vi "Main_State_Calibrate_Position_2.vi"(0 "Motor Position Encoder [deg]":dbl=10.044943820224718 format="%#.3f", 1 "Motor Position Encoder Offset [deg]":dbl caption="Encoder Offset [deg]" format="%#.3f", 5 "Motor Velocity Encoder [deg/s]":dbl format="%#.3f", 7 "Period (Control Loop) [s]":dbl=0.001 caption="Period [s]", 9 "Motor Current Monitor [A]":dbl=-0.009079300589999995, 11 "Requested State":T3, 12 "PID Settings":T1={"Gains"={"K(e)"=0.0, "Kp"=0.8, "Ki"=0.0, "Kd"=0.003}, "Non-linear gain"={"Non-linear gain P"=enum."off", "Non-linear gain I"=enum."off", "Non-linear gain D"=enum."off"}, "D-Part variable"=enum."process variable", "Velocity estimate dy/dt"=enum."external", "Anti reset windup"=TRUE, "I-Part error band"=inf}, 13 "Current Settings":T2={"CW Current Threshold [A]"=0.5, "CCW Current Threshold [A]"=-0.5, "CW Output Range [A]"={"output high"=0.6, "output low"=0.0}, "CCW Output Range [A]"={"output high"=0.0, "output low"=-0.6}}, 14 "Reset?":bool) -> (3 "New Motor Position Encoder Offset [deg]":dbl caption="Encoder Offset [deg]" format="%#.3f", 4 "Velocity Setpoint [deg/s]":dbl, 6 "Command Variable u [A]":dbl, 10 "Calibration Finished?":bool, 15 "New Desired State":T3)   [LabVIEW 2015]
uses:
  Shared TypeDefs/Enum_Robot_States.ctl
  PID_Settings.ctl
  Enum_States_Calibrate_Position.ctl
  <vilib>/addons/control/pid/NI_PID_pid.lvlib
  <vilib>/ptbypt/NI_PtbyPt.lvlib
panel:
  out "Motor Position Encoder ROM CCW [deg]":dbl=10.044943820224718 format="%#_13g"
  out "Motor Position Encoder ROM CW [deg]":dbl=10.044943820224718 format="%#_13g"
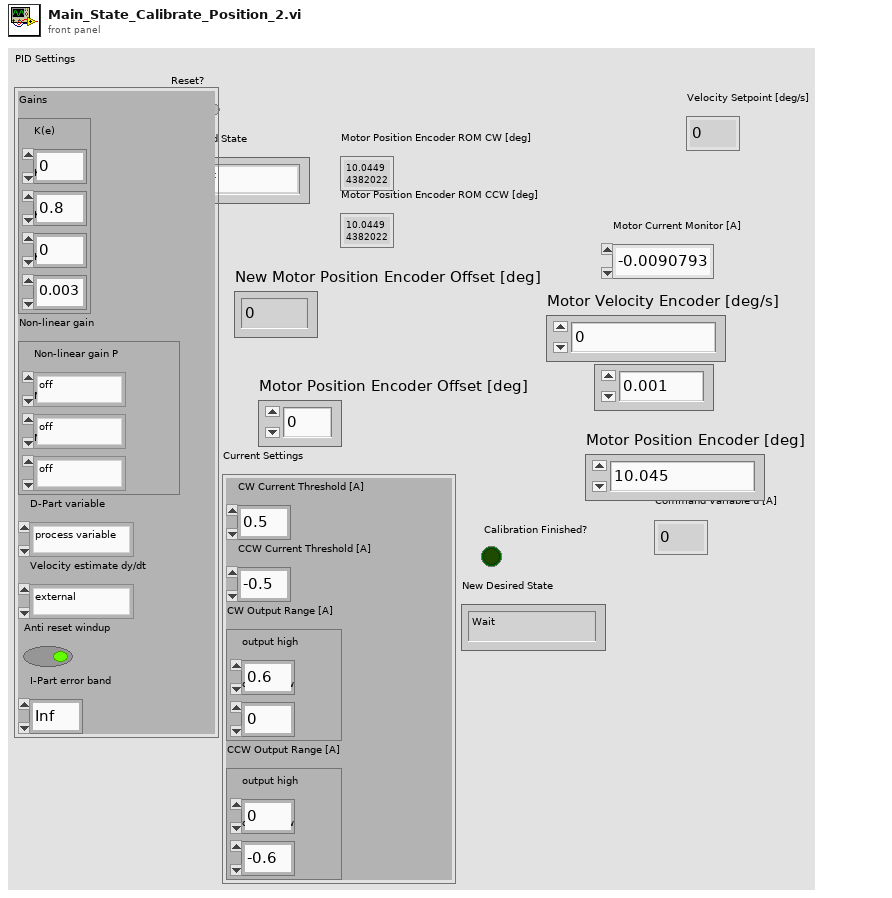
[diagram p1: front panel]
types:
  T1 = typedef "PID_Settings.ctl" = cluster{"Gains":cluster{"K(e)":sgl, "Kp":sgl, "Ki":sgl, "Kd":sgl}, "Non-linear gain":cluster{"Non-linear gain P":enum8{"exponential", "quadratic", "off"}, "Non-linear gain I":enum8{"exponential", "quadratic", "off"}, "Non-linear gain D":enum8{"exponential", "quadratic", "off"}}, "D-Part variable":enum8{"error", "process variable"}, "Velocity estimate dy/dt":enum8{"derivative", "external"}, "Anti reset windup":bool, "I-Part error band":sgl}
  T2 = cluster{"CW Current Threshold [A]":dbl, "CCW Current Threshold [A]":dbl, "CW Output Range [A]":cluster{"output high":dbl, "output low":dbl}, "CCW Output Range [A]":cluster{"output high":dbl, "output low":dbl}}
  T3 = typedef "Enum_Robot_States.ctl" = enum8{"Wait", "Reset", "Calibrate Position", "Calibrate Static Friction", "Hold", "Move (minJerk)", "PID Tuning", "Static Friction Measurement", "Dynamic Friction Measurement"}
  T4 = typedef "Enum_States_Calibrate_Position.ctl" = enum8{"Find Wall CW", "Find Wall CCW"}
  T5 = cluster{"K(e)":sgl, "Kp":sgl, "Ki":sgl, "Kd":sgl}
  T6 = cluster{"Non-linear gain P":enum8{"exponential", "quadratic", "off"}, "Non-linear gain I":enum8{"exponential", "quadratic", "off"}, "Non-linear gain D":enum8{"exponential", "quadratic", "off"}}
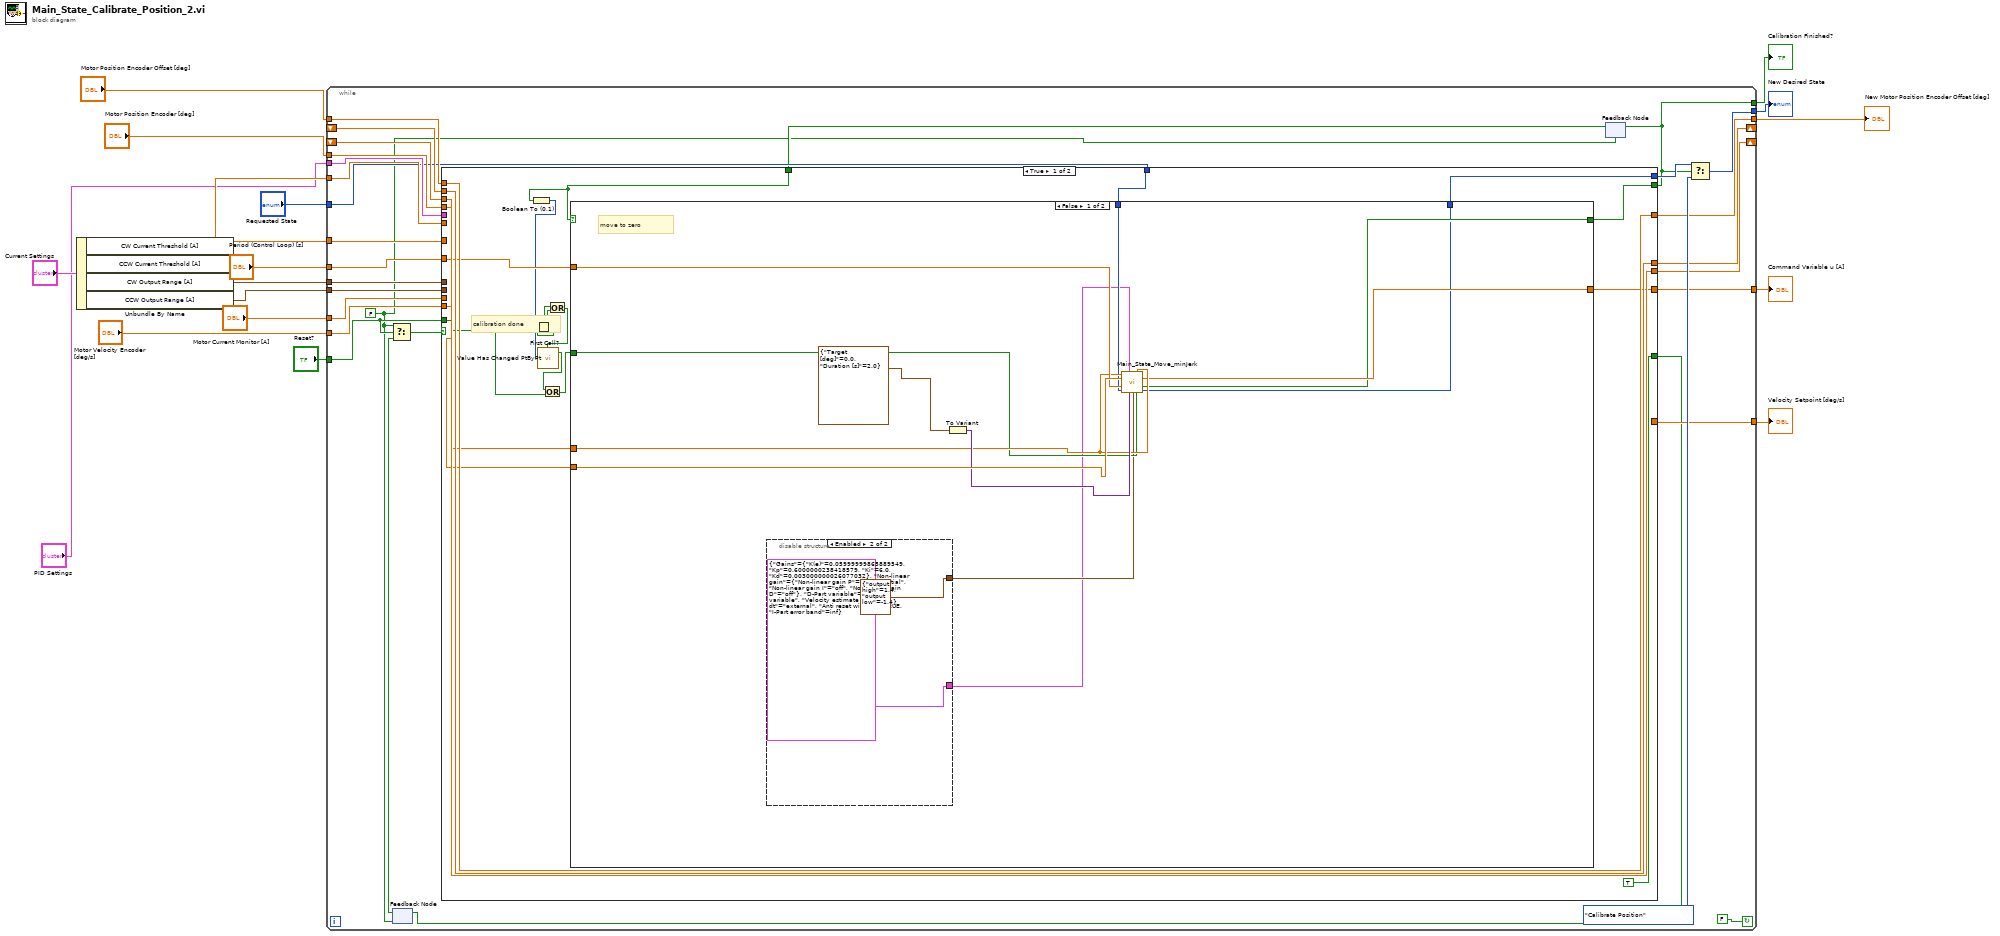
[diagram p0: block diagram]
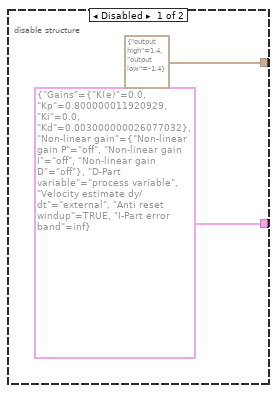
[diagram p2: hidden frame]
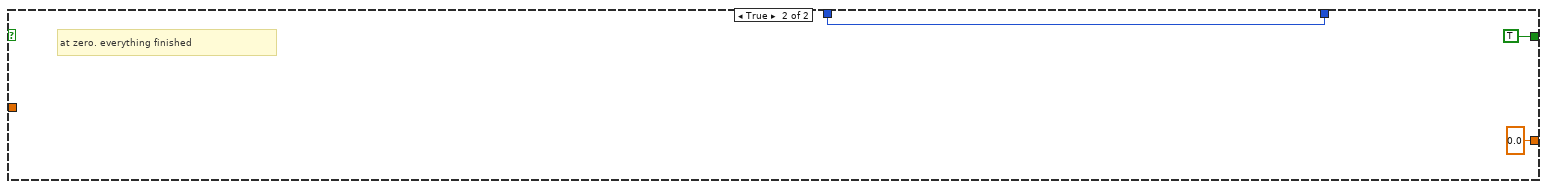
[diagram p3: hidden frame]
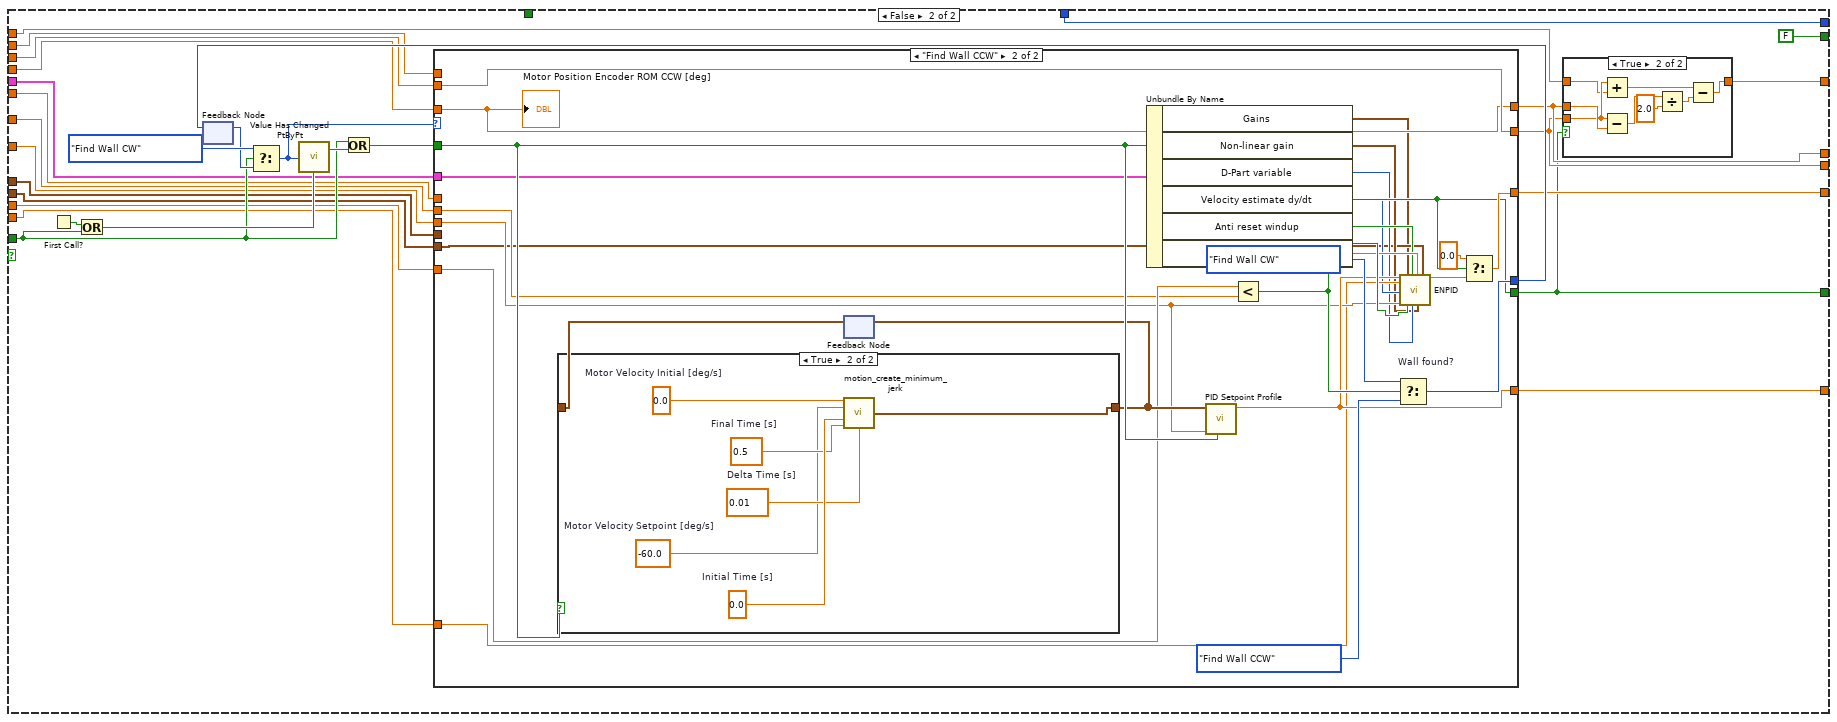
[diagram p4: hidden frame]
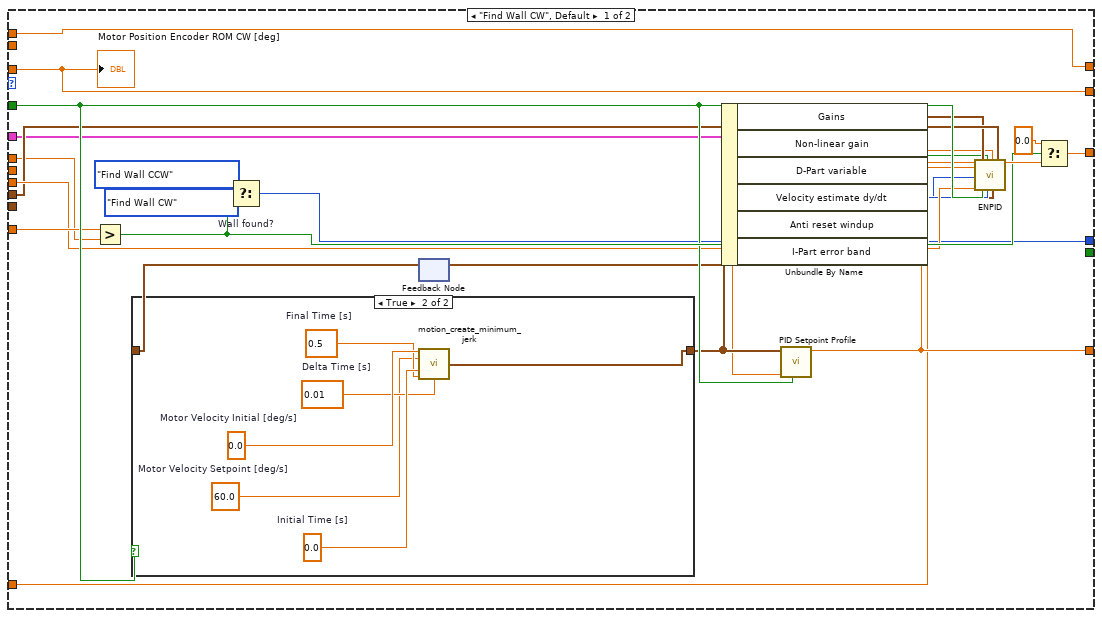
[diagram p6: hidden frame]
diagram:
  n1 = Unbundle By Name("Current Settings") -> ("CW Current Threshold [A]"=w5:dbl, "CCW Current Threshold [A]"=w4:dbl, "CW Output Range [A]"=w3:cluster{"output high":dbl, "output low":dbl}, "CCW Output Range [A]"=w2:cluster{"output high":dbl, "output low":dbl})
  n2 = while {
    tunnel: [w43] -> w18
    tunnel: "Requested State" -> [w23]
    tunnel: [w21] -> w16
    tunnel: [w42] -> w15
    tunnel: [w41] -> w14
    tunnel: "Reset?" -> [w40]
    tunnel: "Motor Current Monitor [A]" -> [w39]
    tunnel: "Period (Control Loop) [s]" -> [w38]
    tunnel: "Motor Velocity Encoder [deg/s]" -> [w37]
    tunnel: "Motor Position Encoder [deg]" -> [w36]
    shift-right: [w35] -> _
    shift-left: _ -> [w34]
    shift-right: [w33] -> _
    shift-left: _ -> [w32]
    tunnel: "Motor Position Encoder Offset [deg]" -> [w31]
    tunnel: [w30] -> w7
    tunnel: w3 -> [w29]
    tunnel: w2 -> [w28]
    tunnel: w4 -> [w27]
    tunnel: w5 -> [w26]
    tunnel: "PID Settings" -> [w25]
    stop <- FALSE continue-if-true
    w19 = FALSE
    n3 = feedback #1(w19) -> (w47:bool)
    n4 = Select(t=w19, s=w40, f=w47) -> (s? t:f=w46:bool)
    n5 = feedback #2(w19) -> (w20:bool)
    n6 = case shown="True" w46 {
      tunnel: [w58 w110] -> w41
      tunnel: w40 -> [w48 w105]
      tunnel: [w55 FALSE] -> w21
      tunnel: [_ w103] -> w42
      tunnel: w39 -> [_ w102]
      tunnel: w38 -> [w59 w101]
      tunnel: w37 -> [w60 w100]
      tunnel: w36 -> [w61 w99]
      tunnel: [w65 w95] -> w35
      tunnel: w34 -> [w65 w98]
      tunnel: [w64 w96] -> w33
      tunnel: w32 -> [w64 w97]
      tunnel: w31 -> [w63 w94]
      tunnel: [w63 w93] -> w30
      tunnel: w29 -> [_ w92]
      tunnel: w28 -> [_ w91]
      tunnel: w27 -> [_ w90]
      tunnel: w26 -> [_ w89]
      tunnel: w25 -> [_ w88]
      tunnel: [TRUE w87] -> w24
      tunnel: w23 -> [w57 w85]
      tunnel: [w56 w85] -> w22
      tunnel: w20 -> [w54 _]
      frame True {
        # "calibration done"
        n7 = Boolean To (0,1)(Boolean=w54) -> (0, 1=w53:i16)
        n8 = First Call?() -> (First Call?: T/F=w52:bool)
        n9 = Or(x=w52, y=w48) -> (x .or. y?=w51:bool)
        n10 = call <vilib>:"Value Has Changed PtByPt.vi"("input data point"=w53, "initialize"=w51) -> ("has changed"=w50:bool)  [unwired: 1 out]
        n11 = Or(x=w50, y=w48) -> (x .or. y?=w49:bool)
        n12 = case shown="False" w54 {
          tunnel: [w72 TRUE] -> w55
          tunnel: w61 -> [w74 _]
          tunnel: w60 -> [w77 _]
          tunnel: w59 -> [w75 _]
          tunnel: [w73 0.0 ("Command Variable u [A]")] -> w58
          tunnel: w57 -> [w71 w83]
          tunnel: [w70 w83] -> w56
          tunnel: w49 -> [w69 _]
          frame False {
            # "move to zero"
            n13 = disable-structure shown="Enabled" {
              disable-tunnel: [cluster{"output high":dbl, "output low":dbl} {"output high"=1.4, "output low"=-1.4} ("Current Settings") cluster{"output high":dbl, "output low":dbl} {"output high"=1.4, "output low"=-1.4} ("Current Settings")] -> w67
              disable-tunnel: [T1 {"Gains"={"K(e)"=0.0, "Kp"=0.8, "Ki"=0.0, "Kd"=0.003}, "Non-linear gain"={"Non-linear gain P"=enum."off", "Non-linear gain I"=enum."off", "Non-linear gain D"=enum."off"}, "D-Part variable"=enum."process variable", "Velocity estimate dy/dt"=enum."external", "Anti reset windup"=TRUE, "I-Part error band"=inf} ("PID Settings") T1 {"Gains"={"K(e)"=0.06, "Kp"=0.6, "Ki"=6.0, "Kd"=0.003}, "Non-linear gain"={"Non-linear gain P"=enum."exponential", "Non-linear gain I"=enum."off", "Non-linear gain D"=enum."off"}, "D-Part variable"=enum."process variable", "Velocity estimate dy/dt"=enum."external", "Anti reset windup"=TRUE, "I-Part error band"=inf} ("PID Settings")] -> w66
              frame Disabled {
              }
              frame Enabled {
              }
            }
            n14 = To Variant(anything=cluster{"Target [deg]":dbl, "Duration [s]":dbl} {"Target [deg]"=0.0, "Duration [s]"=2.0} ("input cluster")) -> (Variant=w76:variant)
            n15 = call "Main_State_Move_minJerk.vi"("Motor Position Encoder [deg]"=w74, "PID Settings"=w66, "Current Settings"=w67, "Initial Setpoint Position [deg]"=w74, "Motor Velocity Encoder [deg/s]"=w77, "Period (Control Loop) [s]"=w75, "Requested State"=w71, "Requested State Details"=w76, "Reset?"=w69) -> ("Command Variable u [A]"=w73:dbl, "Profile Complete?"=w72:bool, "New Desired State"=w70:T3)  [unwired: 2 in, 2 out]
          }
          frame True {
            # "at zero. everything finished"
          }
        }
      }
      frame False {
        w112 = Enum_States_Calibrate_Position."Find Wall CW"
        n16 = First Call?() -> (First Call?: T/F=w109:bool)
        n17 = Or(x=w109, y=w105) -> (x .or. y?=w107:bool)
        n18 = feedback #3(w112) -> (w111:T4)
        n19 = Select(t=w112, s=w105, f=w111) -> (s? t:f=w108:T4)
        n20 = call <vilib>:"Value Has Changed PtByPt.vi"("input data point"=w108, "initialize"=w107) -> ("has changed"=w106:bool)  [unwired: 1 out]
        n21 = Or(x=w105, y=w106) -> (x .or. y?=w104:bool)
        n22 = case shown="\"Find Wall CCW\"" w108 {
          tunnel: [w126 w177] -> w113
          tunnel: [_ w173] -> w87
          tunnel: [w142 w174] -> w110
          tunnel: w104 -> [w141 w172]
          tunnel: [w138 w169] -> w103
          tunnel: w102 -> [w137 w168]
          tunnel: w101 -> [w136 w167]
          tunnel: w100 -> [w135 w166]
          tunnel: w99 -> [w134 w164]
          tunnel: [w134 w165] -> w95
          tunnel: w98 -> [_ w165]
          tunnel: [w133 w164] -> w96
          tunnel: w97 -> [w133 _]
          tunnel: w92 -> [w132 _]
          tunnel: w91 -> [_ w156]
          tunnel: w90 -> [_ w163]
          tunnel: w89 -> [w131 _]
          tunnel: w88 -> [w130 w162]
          frame "Find Wall CW", Default {
            n23 = Greater?(x=w137, y=w131) -> (0:w143:bool)
            n24 = Select "Wall found?"(t=Enum_States_Calibrate_Position."Find Wall CCW", s=w143, f=Enum_States_Calibrate_Position."Find Wall CW") -> (s? t:f=w126:T4)
            n25 = feedback #4() -> (w139:cluster{"time (s)":dbl, "setpoint":dbl}[])  [unwired: 1 in]
            n26 = case shown="True" w141 {
              tunnel: [w148 w150] -> w140
              tunnel: w139 -> [w148 _]
              frame False {
              }
              frame True {
                w149 = 60.0  # Motor Velocity Setpoint [deg/s]
                w151 = 0.01  # Delta Time [s]
                w152 = 0.5  # Final Time [s]
                w153 = 0.0  # Initial Time [s]
                w154 = 0.0  # Motor Velocity Initial [deg/s]
                n27 = call "motion_create_minimum_jerk.vi"("Initial Position"=w154, "Final Position"=w149, "Initial Time [s]"=w153, "Final Time [s]"=w152, "Delta Time [s]"=w151) -> ("Profile"=w150:cluster{"time (s)":dbl, "setpoint":dbl}[])  [unwired: 10 in]
              }
            }
            n28 = feedback-in #4(w140) -> ()
            n29 = Unbundle By Name(w130) -> ("Gains"=w129:T5, "Non-linear gain"=w125:T6, "D-Part variable"=w128:enum8{"error", "process variable"}, "Velocity estimate dy/dt"=w127:enum8{"derivative", "external"}, "Anti reset windup"=w123:bool, "I-Part error band"=w124:sgl)
            n30 = call <vilib>:"PID Setpoint Profile.vi"("reinitialize? (F)"=w141, "dt (s)"=w136, "setpoint profile"=w140) -> ("setpoint"=w138:dbl)  [unwired: 3 in, 3 out]
            n31 = call "ENPID.vi"("r"=w138, "y"=w135, "Velocity estimate dy/dt"=w127, "dt (s)"=w136, "Gains"=w129, "Reset?"=w141, "Anti reset windup"=w123, "D-Part variable"=w128, "I-Part error band"=w124, "Non-linear gain"=w125, "Output range"=w132) -> ("u"=w145:dbl)  [unwired: 7 in, 1 out]
            n32 = Select(t=0.0, s=w143, f=w145) -> (s? t:f=w142:dbl)
            "Motor Position Encoder ROM CW [deg]" <- w134
          }
          frame "Find Wall CCW" {
            n33 = feedback #5() -> (w170:cluster{"time (s)":dbl, "setpoint":dbl}[])  [unwired: 1 in]
            n34 = case shown="True" w172 {
              tunnel: [w180 w186] -> w171
              tunnel: w170 -> [w180 _]
              frame False {
              }
              frame True {
                w181 = -60.0  # Motor Velocity Setpoint [deg/s]
                w182 = 0.01  # Delta Time [s]
                w183 = 0.5  # Final Time [s]
                w184 = 0.0  # Initial Time [s]
                w185 = 0.0  # Motor Velocity Initial [deg/s]
                n35 = call "motion_create_minimum_jerk.vi"("Initial Position"=w185, "Final Position"=w181, "Initial Time [s]"=w184, "Final Time [s]"=w183, "Delta Time [s]"=w182) -> ("Profile"=w186:cluster{"time (s)":dbl, "setpoint":dbl}[])  [unwired: 10 in]
              }
            }
            n36 = feedback-in #5(w171) -> ()
            n37 = Unbundle By Name(w162) -> ("Gains"=w155:T5, "Non-linear gain"=w157:T6, "D-Part variable"=w158:enum8{"error", "process variable"}, "Velocity estimate dy/dt"=w159:enum8{"derivative", "external"}, "Anti reset windup"=w160:bool, "I-Part error band"=w161:sgl)
            n38 = call <vilib>:"PID Setpoint Profile.vi"("reinitialize? (F)"=w172, "dt (s)"=w167, "setpoint profile"=w171) -> ("setpoint"=w169:dbl)  [unwired: 3 in, 3 out]
            n39 = Less?(x=w168, y=w163) -> (x < y?=w173:bool)
            n40 = Select "Wall found?"(t=Enum_States_Calibrate_Position."Find Wall CW", s=w173, f=Enum_States_Calibrate_Position."Find Wall CCW") -> (s? t:f=w177:T4)
            n41 = call "ENPID.vi"("r"=w169, "y"=w166, "Velocity estimate dy/dt"=w159, "dt (s)"=w167, "Gains"=w155, "Reset?"=w172, "Anti reset windup"=w160, "D-Part variable"=w158, "I-Part error band"=w161, "Non-linear gain"=w157, "Output range"=w156) -> ("u"=w175:dbl)  [unwired: 7 in, 1 out]
            n42 = Select(t=0.0, s=w173, f=w175) -> (s? t:f=w174:dbl)
            "Motor Position Encoder ROM CCW [deg]" <- w164
          }
        }
        n43 = feedback-in #3(w113) -> ()
        n44 = case shown="True" w87 {
          tunnel: w96 -> [_ w118]
          tunnel: w95 -> [_ w117]
          tunnel: w94 -> [w114 w116]
          tunnel: [w114 w115] -> w93
          frame False {
          }
          frame True {
            n45 = Add(x=w117, y=w116) -> (x+y=w119:dbl)
            n46 = Subtract(x=w117, y=w118) -> (x-y=w122:dbl)
            n47 = Divide(x=w122, y=2.0) -> (x/y=w120:dbl)
            n48 = Subtract(x=w119, y=w120) -> (x-y=w115:dbl)
          }
        }
      }
    }
    n49 = feedback-in #1(w24) -> ()
    n50 = feedback-in #2(w21) -> ()
    n51 = Select(t=w22, s=w21, f=Enum_Robot_States."Calibrate Position") -> (s? t:f=w43:T3)
  }
  "New Desired State" <- w18
  "Calibration Finished?" <- w16
  "Velocity Setpoint [deg/s]" <- w15
  "Command Variable u [A]" <- w14
  "New Motor Position Encoder Offset [deg]" <- w7
